vi "Set Aout Limit Error.vi"(8 "error in (no error)":errorcluster, 9 "firmware revision":string(combo), 10 "aout limit error":T1, 11 "VISA resource name":refnum<visa-resource-name>) -> (0 "error out":errorcluster, 2 "bridge error":T2, 3 "VISA resource name out":refnum<visa-resource-name>)   [LabVIEW 2025, in "Andeen-Hagerling 2700A.lvlib"]
doc: "The analog outputs levels for the capacitance and loss channels\nmay not exceed the upper and lower voltage protection\nlimits. This VI is used to enable and disable the error\nreporting associated with this voltage clipping capability."
uses:
  Andeen-Hagerling 2700A.lvlib
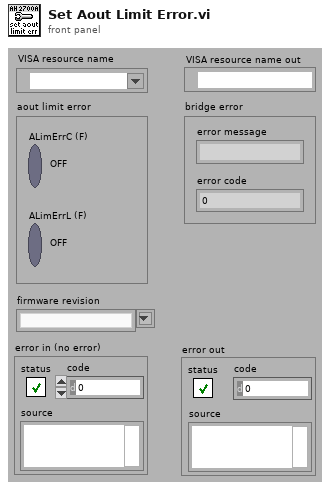
[diagram p1: front panel]
types:
  T1 = cluster{"ALimErrC (F)":bool, "ALimErrL (F)":bool}
  T2 = cluster{"error message":string, "error code":i32}
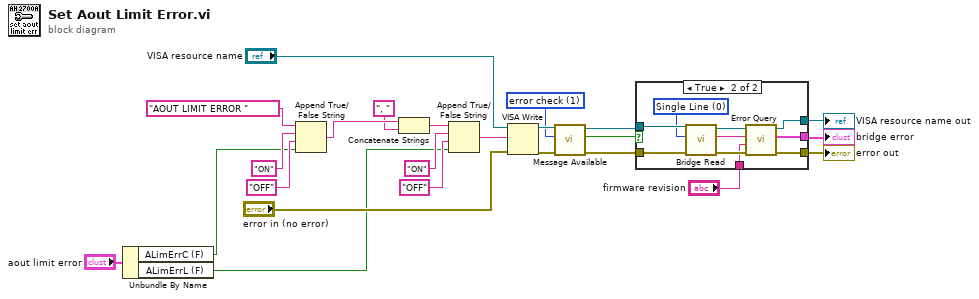
[diagram p0: block diagram]
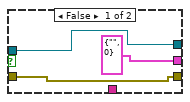
[diagram p2: hidden frame]
diagram:
  w1 = u16 1 items=["none", "error check", "multiline read", "infinite"] ("delay")
  n1 = Unbundle By Name("aout limit error") -> ("ALimErrC (F)"=w3:bool, "ALimErrL (F)"=w2:bool)
  n2 = Append True/False String(1:w3, 2:"OFF" ("false string"), 3:"ON" ("true string"), 4:"AOUT LIMIT ERROR " ("command")) -> (0:w21:string)
  n3 = Concatenate Strings(w21, ", " ("command")) -> (w15:string)
  n4 = Append True/False String(1:w2, 2:"OFF" ("false string"), 3:"ON" ("true string"), 4:w15) -> (0:w16:string)
  n5 = VISA Write(VISA resource name="VISA resource name", write buffer=w16, error in (no error)="error in (no error)") -> (VISA resource name out=w9:refnum<visa-resource-name>, error out=w8:errorcluster)  [unwired: 1 out]
  n6 = call "Message Available.vi"("error in (no error)"=w8, "delay"=w1, "VISA resource name"=w9) -> ("error out"=w11:errorcluster, "message available"=w13:bool, "VISA resource name out"=w12:refnum<visa-resource-name>)  [unwired: 6 in]
  n7 = case shown="True" w13 {
    tunnel: w12 -> [w26 w34]
    tunnel: w11 -> [w27 w33]
    tunnel: "firmware revision" -> [_ w32]
    tunnel: [w27 w31] -> w7
    tunnel: [w26 w30] -> w5
    tunnel: [T2 {"error message"="", "error code"=0} ("bridge error") w29] -> w6
    frame False {
    }
    frame True {
      w28 = u16 0 items=["Single Line", "Multi-Line"] ("Multiline")
      n8 = call "Bridge Read.vi"("error in (no error)"=w33, "multiline"=w28, "VISA resource name"=w34) -> ("error out"=w36:errorcluster, "read buffer"=w37:string, "VISA resource name out"=w35:refnum<visa-resource-name>)  [unwired: 6 in]
      n9 = call "Error Query.vi"("error in (no error)"=w36, "firmware revision"=w32, "measurement line"=w37, "VISA resource name"=w35) -> ("error out"=w31:errorcluster, "bridge error"=w29:T2, "VISA resource name out"=w30:refnum<visa-resource-name>)  [unwired: 5 in]
    }
  }
  "VISA resource name out" <- w5
  "error out" <- w7
  "bridge error" <- w6
